vi "Create Loc String Object.vi"(10 "error in (no error)":errorcluster, 11 "Name":string) -> (2 "error out":errorcluster, 3 ".NET Refnum out":refnum<k24>)   [LabVIEW 2015, in "Configuration Tool.lvlib"]
uses:
  Configuration Tool.lvlib
  NationalInstruments.VeriStand.XMLReader
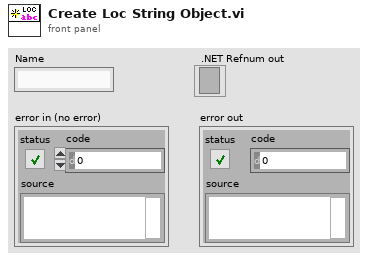
[diagram p1: front panel]
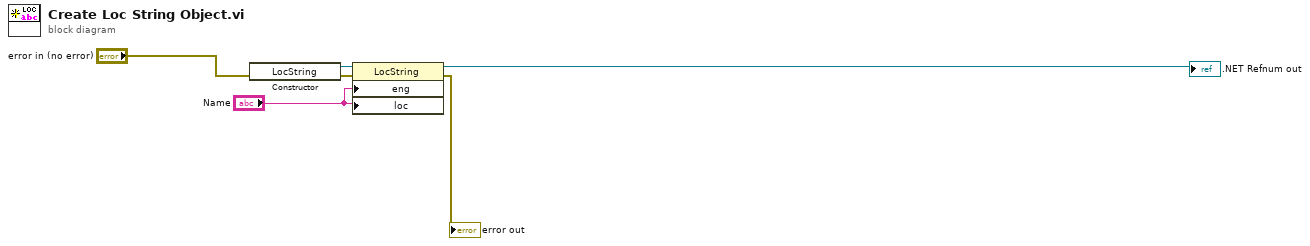
[diagram p0: block diagram]
diagram:
  n1 = constructor class="LocString"(error in="error in (no error)") -> (reference out=w5:refnum<k24>, error out=w6:errorcluster)  [unwired: 2 in, 1 out]
  n2 = property class="LocString"(reference=w5, error in=w6, "eng"="Name", "loc"="Name") -> (reference out=→".NET Refnum out":refnum<k24>, error out=→"error out":errorcluster)
